vi "TAI_Servo.vi"(3 "Normal Output":dbl, 4 "Aux Trigger":bool, 5 "Override Actuator Bypass":bool, 6 "Actuator Name":string) -> (0 "Interlocked Output":dbl, 2 "Output Mode":T1(ring))   [LabVIEW 2020]
doc: "This VI is configured for polymorphic use and functions as an interlock, allowing the selected servo to be tested manually via the FRC 4265 Dashboard. During testing, all interlocked actuators which are not selected for testing are disabled."
uses:
  cf260dee-87cd-4ad6-a0e3-c3116b7c1a2f.vi
  e00df7bd-b999-461d-9362-47e176d3d7d1.vi
  GlobalDriverStationData.vi
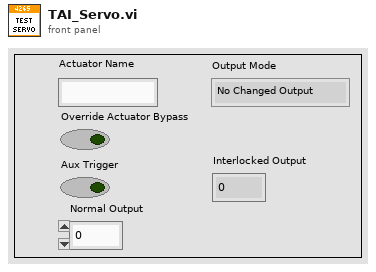
[diagram p1: front panel]
types:
  T1 = enum16{"No Changed Output", "New Normal Output", "New Testing Output"}
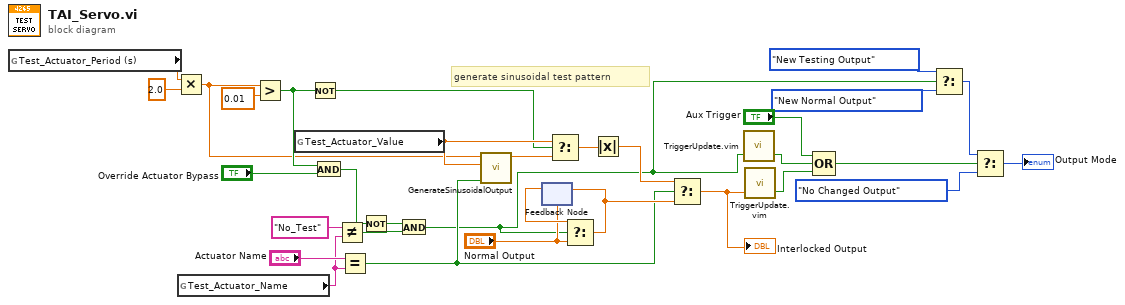
[diagram p0: block diagram]
diagram:
  # "generate sinusoidal test pattern"
  n1 = global read "GlobalDriverStationData.vi" "Test_Actuator_Period (s)"() -> (w15:dbl)
  n2 = Multiply(x=w15, y=2.0) -> (x*y=w14:dbl)
  n3 = global read "GlobalDriverStationData.vi" "Test_Actuator_Name"() -> (w30:string)
  n4 = Greater?(x=w14, y=0.01) -> (0:w18:bool)
  n5 = global read "GlobalDriverStationData.vi" "Test_Actuator_Value"() -> (w25:dbl)
  n6 = Not(x=w18) -> (.not. x?=w13:bool)
  n7 = And(x=w18, y="Override Actuator Bypass") -> (x .and. y?=w21:bool)
  n8 = Not Equal?(x="No_Test", y=w30) -> (x != y?=w19:bool)
  n9 = Equal?(x="Actuator Name", y=w30) -> (x = y?=w3:bool)
  n10 = Not(x=w21) -> (.not. x?=w20:bool)
  n11 = And(x=w20, y=w19) -> (x .and. y?=w2:bool)
  n12 = call "GenerateSinusoidalOutput.vi"("Init"=w3, "Amplitude"=w25, "Period (s)"=w14) -> ("sin(time)"=w26:dbl)  [unwired: 8 in]
  n13 = feedback #1("Normal Output") -> (w29:dbl)
  n14 = Select(t=w25, s=w13, f=w26) -> (s? t:f=w24:dbl)
  n15 = Select(t=w29, s=w2, f="Normal Output") -> (s? t:f=w27:dbl)
  n16 = feedback-in #1(w27) -> ()
  n17 = Absolute Value(x=w24) -> (abs(x)=w17:dbl)
  n18 = Select(t=w17, s=w3, f=w27) -> (s? t:f=w7:dbl)
  "Interlocked Output" <- w7
  n19 = call "TriggerUpdate.vim"("Trigger"=w2) -> ("Update"=w6:bool)  [unwired: 2 in]
  n20 = call "TriggerUpdate.vim"("Trigger"=w7) -> ("Update"=w5:bool)  [unwired: 2 in]
  n21 = Compound Arithmetic op=OR("Aux Trigger", w6, w5) -> (w4:bool)
  n22 = Select(t=T1."New Testing Output", s=w2, f=T1."New Normal Output") -> (s? t:f=w10:T1)
  n23 = Select(t=w10, s=w4, f=T1."No Changed Output") -> (s? t:f=→"Output Mode":T1)
